vi "SDSU_MemLocsMngr.vi"(7 "action":enum16{"set", "get", "clear", "getall"}(ring)=enum."get", 8 "value":u32, 9 "address":i32 format="%x", 10 "type":string, 11 "board":i32) -> (1 "array":T1[](array[typedef]) {"address" format="%x"}, 2 "found":bool)   [LabVIEW 2016]
uses:
  SDSU_MemLoc.ctl
panel:
  in  "location":T1 {"address" format="%x"}
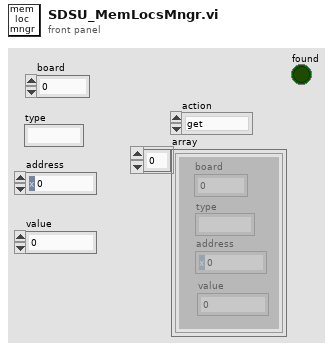
[diagram p1: front panel]
types:
  T1 = typedef "SDSU_MemLoc.ctl" = cluster{"board":i32, "type":string, "address":i32, "value":u32}
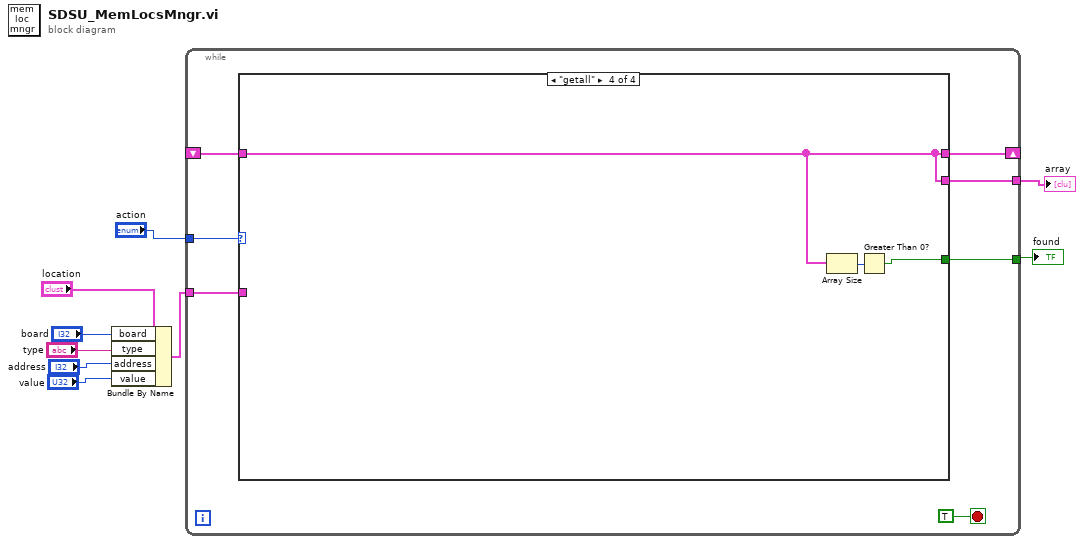
[diagram p0: block diagram]
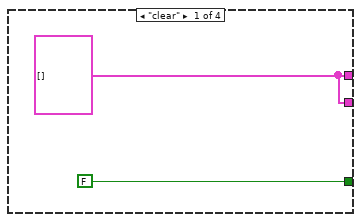
[diagram p2: hidden frame]
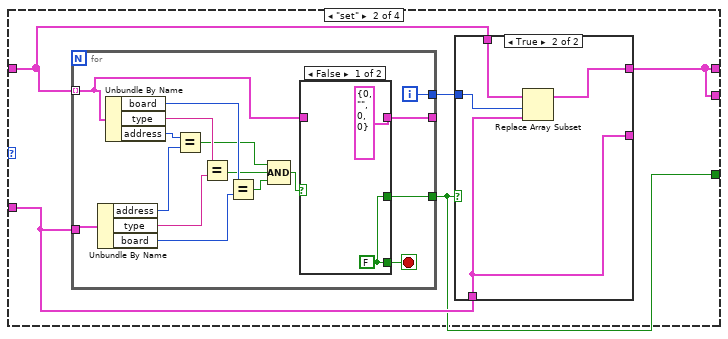
[diagram p3: hidden frame]
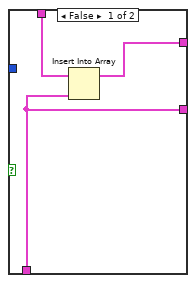
[diagram p4: hidden frame]
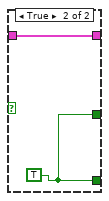
[diagram p5: hidden frame]
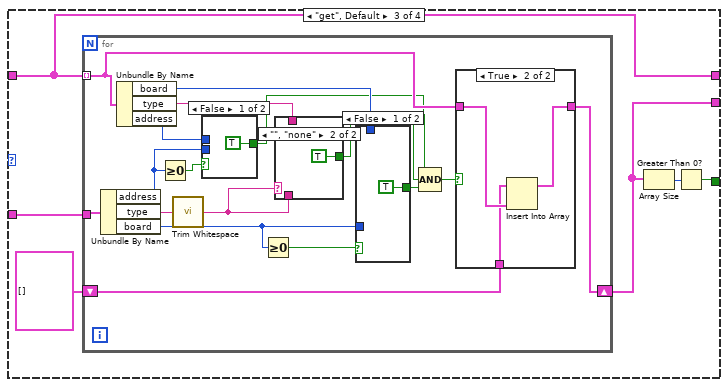
[diagram p6: hidden frame]
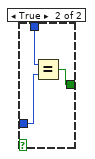
[diagram p7: hidden frame]
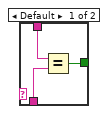
[diagram p8: hidden frame]
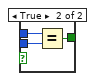
[diagram p9: hidden frame]
diagram:
  n1 = Bundle By Name(cluster="location", "board"="board", "type"="type", "address"="address", "value"="value") -> (w6:T1)
  n2 = while {
    tunnel: "action" -> [w15]
    shift-right: [w13] -> _
    shift-left: _ -> [w12]
    tunnel: w6 -> [w14]
    tunnel: [w11] -> w1
    tunnel: [w10] -> w8
    stop <- TRUE stop-if-true
    n3 = case shown="\"getall\"" w15 {
      tunnel: w14 -> [_ w22 w56 _]
      tunnel: [w17 w19 w55 w91] -> w13
      tunnel: w12 -> [_ w23 w55 w91]
      tunnel: [w17 w19 w53 w91] -> w11
      tunnel: [FALSE w21 w52 w90] -> w10
      frame "clear" {
        w17 = T1[] []
      }
      frame "set" {
        n4 = for {
          tunnel: w23 -> [w39] mode=indexing
          tunnel: w22 -> [w46]
          tunnel: [w37] -> _
          tunnel: [w36] -> w21
          tunnel: [w35] -> w20
          i -> [w35]
          stop <- w38 stop-if-true
          n5 = Unbundle By Name(w46) -> ("address"=w44:i32, "type"=w42:string, "board"=w40:i32)
          n6 = Unbundle By Name(w39) -> ("board"=w41:i32, "type"=w43:string, "address"=w45:i32)
          n7 = Equal?(x=w45, y=w44) -> (x = y?=w32:bool)
          n8 = Equal?(x=w43, y=w42) -> (x = y?=w33:bool)
          n9 = Equal?(x=w41, y=w40) -> (x = y?=w34:bool)
          n10 = Compound Arithmetic op=AND(w32, w33, w34) -> (w31:bool)
          n11 = case shown="False" w31 {
            tunnel: w39 -> [_ w50]
            tunnel: [w48 w49] -> w38
            tunnel: [T1 {"board"=0, "type"="", "address"=0, "value"=0} ("location") w50] -> w37
            tunnel: [w48 w49] -> w36
            frame False {
              w48 = FALSE
            }
            frame True {
              w49 = TRUE
            }
          }
        }
        n12 = case shown="True" w21 {
          tunnel: [w26 w29] -> w19
          tunnel: w23 -> [w25 w30]
          tunnel: w22 -> [w24 w27]
          tunnel: [w24 w27] -> _
          tunnel: w20 -> [_ w28]
          frame False {
            n13 = Insert Into Array(array=w25, new element=w24) -> (w26:T1[])  [unwired: 1 in]
          }
          frame True {
            n14 = Replace Array Subset(array=w30, new element=w27, index=w28) -> (w29:T1[])
          }
        }
      }
      frame "get", Default {
        n15 = for {
          tunnel: w55 -> [w68] mode=indexing
          tunnel: w56 -> [w73]
          shift-right: [w58] -> w53
          shift-left: T1[] [] -> [w57]
          n16 = Unbundle By Name(w73) -> ("address"=w66:i32, "type"=w70:string, "board"=w64:i32)
          n17 = Unbundle By Name(w68) -> ("board"=w69:i32, "type"=w71:string, "address"=w72:i32)
          n18 = Greater Or Equal To 0?(x=w66) -> (x >= 0?=w67:bool)
          n19 = call <vilib>:"Trim Whitespace.vi"("string"=w70) -> ("trimmed string"=w65:string)  [unwired: 1 in]
          n20 = case shown="False" w67 {
            tunnel: w72 -> [_ w85]
            tunnel: w66 -> [_ w84]
            tunnel: [TRUE w83] -> w59
            frame False {
            }
            frame True {
              n21 = Equal?(x=w85, y=w84) -> (x = y?=w83:bool)
            }
          }
          n22 = Greater Or Equal To 0?(x=w64) -> (x >= 0?=w63:bool)
          n23 = case shown="\"\", \"none\"" w65 {
            tunnel: w71 -> [w80 _]
            tunnel: w65 -> [w79 _]
            tunnel: [w78 TRUE] -> w60
            frame Default {
              n24 = Equal?(x=w80, y=w79) -> (x = y?=w78:bool)
            }
            frame "", "none" {
            }
          }
          n25 = case shown="False" w63 {
            tunnel: w69 -> [_ w77]
            tunnel: w64 -> [_ w76]
            tunnel: [TRUE w75] -> w62
            frame False {
            }
            frame True {
              n26 = Equal?(x=w77, y=w76) -> (x = y?=w75:bool)
            }
          }
          n27 = Compound Arithmetic op=AND(w59, w60, w62) -> (w61:bool)
          n28 = case shown="True" w61 {
            tunnel: w68 -> [_ w89]
            tunnel: [w86 w88] -> w58
            tunnel: w57 -> [w86 w87]
            frame False {
            }
            frame True {
              n29 = Insert Into Array(array=w87, new element=w89) -> (w88:T1[])  [unwired: 1 in]
            }
          }
        }
        n30 = Array Size(array=w53) -> (size(s)=w51:i32)
        n31 = Greater Than 0?(x=w51) -> (x > 0?=w52:bool)
      }
      frame "getall" {
        n32 = Array Size(array=w91) -> (size(s)=w92:i32)
        n33 = Greater Than 0?(x=w92) -> (x > 0?=w90:bool)
      }
    }
  }
  "found" <- w8
  "array" <- w1
